vi "Init Editor Panels.vi"(8 "PanelArray in":refnum<class "ArrayManager.lvclass">, 9 "Types":T1[](array[typedef]), 10 "Is Worker Variant?":bool, 11 "Worker lvlib":path) -> (0 "error out":errorcluster, 4 "Failed Value Editors":string[](array[string]))   [LabVIEW 2020, in "FlexBlocks.lvlib"]
uses:
  FlexBlocks.lvlib
  Type Descriptor.ctl
  Terminal Direction.ctl
  Value Mode.ctl
  Special Terminal.ctl
  <vilib>/IlluminatedG/IG OOPanel/OOPanel/ArrayManager/ArrayManager.lvclass
  Terminal Mode.ctl
  Value Editor Base/Value Editor Base.lvclass
  C:/Program Files (x86)/National Instruments/LabVIEW 2020/vi.lib/IlluminatedG/IG OOPanel/OOPanel/ArrayPanel/ArrayPanel.lvclass
  C:/Program Files (x86)/National Instruments/LabVIEW 2020/vi.lib/IlluminatedG/IG OOPanel/OOPanel/Panel/Panel.lvclass
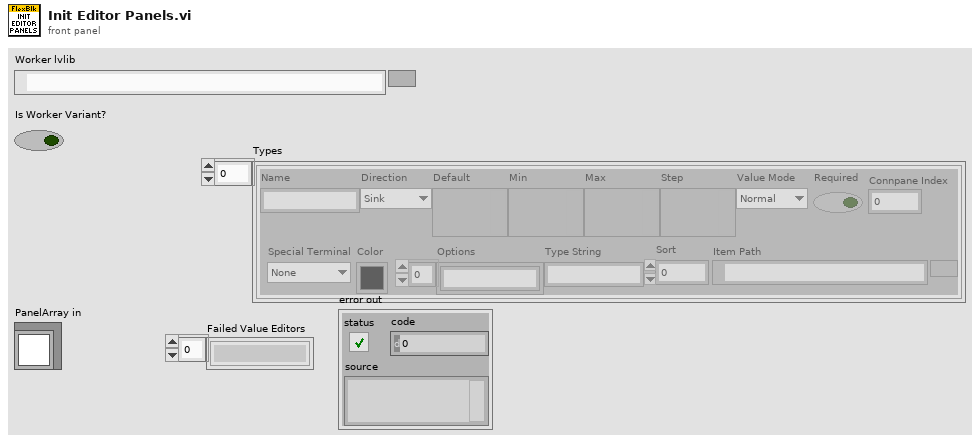
[diagram p1: front panel]
types:
  T1 = typedef "FlexBlocks.lvlib/Type Descriptor.ctl" = cluster{"Name":string, "Direction":T2, "Default":variant, "Min":variant, "Max":variant, "Step":variant, "Value Mode":T3, "Required":bool, "Connpane Index":i32, "Special Terminal":T4, "Color":u32, "Options":string[], "Type String":string, "Sort":i32, "Item Path":path}
  T2 = typedef "FlexBlocks.lvlib/Terminal Direction.ctl" = enum16{"Sink", "Source"}
  T3 = typedef "FlexBlocks.lvlib/Value Mode.ctl" = enum16{"Normal", "Range", "Select"}
  T4 = typedef "FlexBlocks.lvlib/Special Terminal.ctl" = enum16{"None", "Action", "Init", "Tag", "State in", "State out", "Error"}
  T5 = map{string, refnum<class "Value Editor Base.lvclass">}
  T6 = typedef "FlexBlocks.lvlib/Terminal Mode.ctl" = enum16{"Channel", "Config", "Value", "Control Ref"}
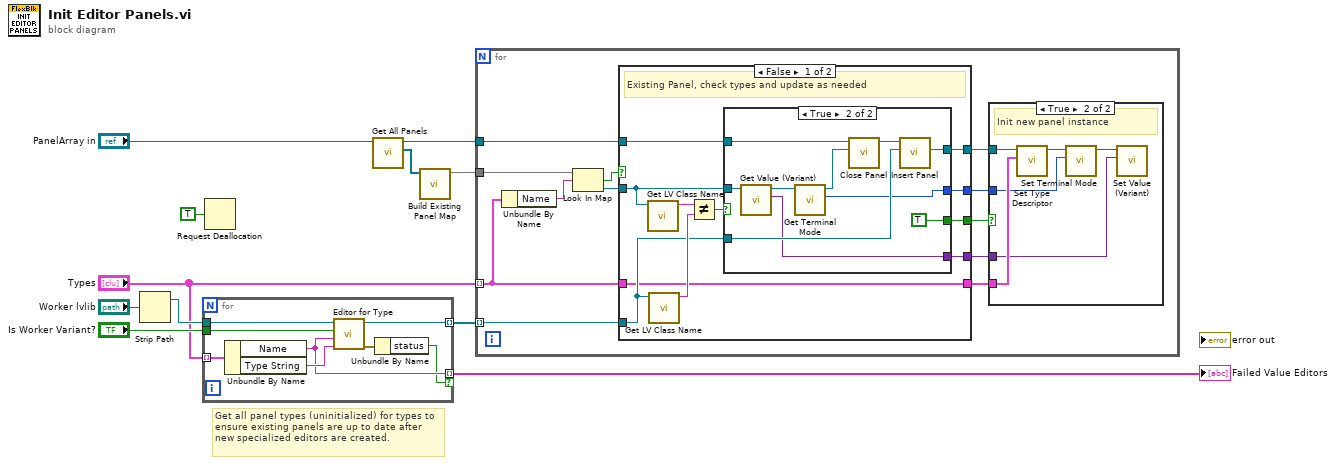
[diagram p0: block diagram]
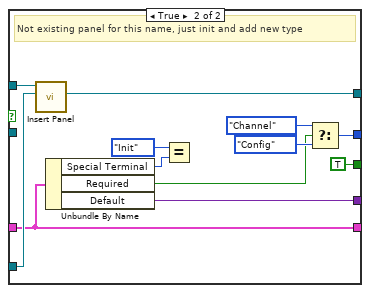
[diagram p3: hidden frame]
diagram:
  # "Get all panel types (uninitialized) for types to ensure existing panels are up to date after new specialized editors are created."
  n1 = Strip Path(path="Worker lvlib") -> (stripped path=w9:path)  [unwired: 1 out]
  n2 = for {
    tunnel: "Is Worker Variant?" -> [w17]
    tunnel: w9 -> [w18]
    tunnel: "Types" -> [w19] mode=indexing
    tunnel: [w15] -> w6 mode=indexing if=w13
    tunnel: [w12] -> w5 mode=indexing
    n3 = Unbundle By Name(w19) -> ("Name"=w15:string, "Type String"=w16:string)
    n4 = call "Editor for Type.vi"("Value Type String"=w16, "Value Name"=w15, "Is Variant"=w17, "Worker/Variant Folder"=w18) -> ("error out"=w14:errorcluster, "Value Editor"=w12:refnum<class "Value Editor Base.lvclass">)  [unwired: 6 in]
    n5 = Unbundle By Name(w14) -> ("status"=w13:bool)
  }
  "Failed Value Editors" <- w6
  n6 = Request Deallocation(TRUE ("flag")) -> ()
  n7 = call <vilib>:"Get All Panels.vi"("PanelArray in"="PanelArray in") -> ("Panels"=w7:refnum<class "ArrayPanel.lvclass">[], "PanelArray out"=w2:refnum<class "ArrayManager.lvclass">)  [unwired: 8 in, 1 out]
  n8 = call "Build Existing Panel Map.vi"("Panels"=w7) -> ("Existing Panel Map"=w3:T5)  [unwired: 10 in]
  n9 = for {
    tunnel: w5 -> [w26] mode=indexing
    tunnel: "Types" -> [w25] mode=indexing
    tunnel: w3 -> [w31]
    tunnel: w2 -> [w27]
    n10 = Unbundle By Name(w25) -> ("Name"=w30:string)
    n11 = Look In Map(map=w31, key=w30) -> (key not found?=w29:bool, value=w28:refnum<class "Value Editor Base.lvclass">)  [unwired: 1 in]
    n12 = case shown="False" w29 {
      tunnel: w28 -> [w39 _]
      tunnel: w27 -> [w38 w64]
      tunnel: w26 -> [w37 w63]
      tunnel: w25 -> [w33 w59]
      tunnel: [w36 w62] -> w24
      tunnel: [w35 TRUE] -> w22
      tunnel: [w34 w61] -> w23
      tunnel: [w33 w59] -> w21
      tunnel: [w32 w55] -> w20
      frame False {
        # "Existing Panel, check types and update as needed"
        n13 = call <vilib>:"Get LV Class Name.vi"("object"=w39) -> ("class name"=w42:string)  [unwired: 9 in, 1 out]
        n14 = call <vilib>:"Get LV Class Name.vi"("object"=w37) -> ("class name"=w41:string)  [unwired: 9 in, 1 out]
        n15 = Not Equal?(x=w42, y=w41) -> (x != y?=w40:bool)
        n16 = case shown="True" w40 {
          tunnel: w39 -> [_ w52]
          tunnel: w38 -> [_ w47]
          tunnel: w37 -> [_ w51]
          tunnel: [_ w50] -> w34
          tunnel: [_ TRUE] -> w35
          tunnel: [_ w48] -> w36
          tunnel: [_ w43] -> w32
          frame False {
            # "Still good, no changes"
          }
          frame True {
            n17 = call "Get Value (Variant).vi"("Value Editor Base in"=w52) -> ("Value"=w50:variant, "Value Editor Base out"=w45:refnum<class "Value Editor Base.lvclass">)  [unwired: 8 in, 1 out]
            n18 = call "Get Terminal Mode.vi"("Value Editor Base in"=w45) -> ("Terminal Mode"=w43:T6, "Value Editor Base out"=w44:refnum<class "Value Editor Base.lvclass">)  [unwired: 8 in, 1 out]
            n19 = call <vilib>:"Close Panel.vi"("ArrayPanel"=w44, "ArrayManager in"=w47) -> ("ArrayManager in"=w46:refnum<class "ArrayManager.lvclass">)  [unwired: 8 in, 1 out]
            n20 = call <vilib>:"Insert Panel.vi"("Panel/Type"=w51, "PanelArray in"=w46) -> ("Panel/Type"=w48:refnum<class "Value Editor Base.lvclass">)  [unwired: 7 in, 2 out]
          }
        }
      }
      frame True {
        # "Not existing panel for this name, just init and add new type"
        n21 = call <vilib>:"Insert Panel.vi"("Panel/Type"=w63, "PanelArray in"=w64) -> ("Panel/Type"=w62:refnum<class "Value Editor Base.lvclass">)  [unwired: 7 in, 2 out]
        n22 = Unbundle By Name(w59) -> ("Special Terminal"=w58:T4, "Required"=w54:bool, "Default"=w61:variant)
        n23 = Equal?(x=Special_Terminal."Init", y=w58) -> ()  [unwired: 1 out]
        n24 = Select(t=Terminal_Mode."Channel" ("Terminal Mode"), s=w54, f=Terminal_Mode."Config" ("Terminal Mode")) -> (s? t:f=w55:T6)
      }
    }
    n25 = case shown="True" w22 {
      tunnel: w24 -> [_ w70]
      tunnel: w23 -> [_ w65]
      tunnel: w21 -> [_ w69]
      tunnel: w20 -> [_ w67]
      frame False {
      }
      frame True {
        # "Init new panel instance"
        n26 = call "Set Type Descriptor.vi"("Type Descriptor"=w69, "Value Editor Base in"=w70) -> ("Value Editor Base out"=w68:refnum<class "Value Editor Base.lvclass">)  [unwired: 8 in, 1 out]
        n27 = call "Set Terminal Mode.vi"("Terminal Mode"=w67, "Value Editor Base in"=w68) -> ("Value Editor Base out"=w66:refnum<class "Value Editor Base.lvclass">)  [unwired: 8 in, 1 out]
        n28 = call "Set Value (Variant).vi"("Value"=w65, "Value Editor Base in"=w66) -> ()  [unwired: 8 in, 2 out]
      }
    }
  }
